vi "Quick Scale 1D.vi"(0 "X":dbl[](array[numeric]) format="%0.2f") -> (1 "Y[i]=X[i]/Max|X|":dbl[](array[numeric]) format="%0.2f", 2 "max|X|":dbl format="%0.2f", 3 "error":i32)   [LabVIEW 2020, in "NI_AALBase.lvlib"]
doc: "Determines the maximum absolute value of the input <B>X</B> and then scales <B>X</B> using this value."
uses:
  <vilib>/Analysis/NI_AALBase.lvlib
  <resource>/lvanlys.dll
panel:
  # "Y[i]=X[i]/Max|X|"
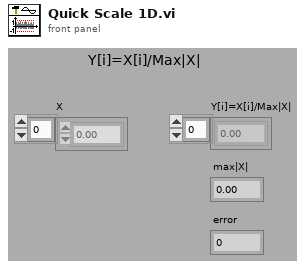
[diagram p1: front panel]
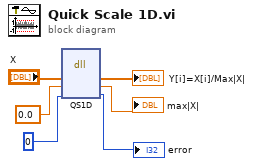
[diagram p0: block diagram]
diagram:
  n1 = dll-call lib="e:/builds/penguin/labview/branches/2020/dev/dist/resource/lvanlys.*" fn="QS1D"("X"="X", "output param"=0.0, "output param"=0) -> ("X"=→"Y[i]=X[i]/Max|X|":dbl[], "output param"=→"max|X|":dbl, "output param"=→"error":i32)  [unwired: 4 in, 2 out]
